vi "Begin.vi"(11 "Image Size":T1=enum."320x240") -> (0 "error out":errorcluster)   [LabVIEW 2012]
doc: "Called before other user functions, this VI is expected to open initial I/O refnums, load in file data, and do all program initialization. Notice that the <B>error out</B> terminal is simply used for data flow. Wiring it to other structures or subVIs ensures that this VI runs first."
uses:
  <vilib>/Rock Robotics/WPI/Camera/WPI_CameraImageSize.ctl
  <vilib>/Rock Robotics/WPI/DriverStation/WPI_DriverStationRobotMode2.ctl
  <vilib>/Rock Robotics/SystemInterfaces/DIO/FPGA_DIOPWMChannel.ctl
  <vilib>/Rock Robotics/WPI/Joystick/WPI_JoystickDeviceEnum.ctl
  <vilib>/Rock Robotics/SystemInterfaces/Typedef/FPGA_TypedefDigitalModule.ctl
  <vilib>/Rock Robotics/WPI/Relay/WPI_RelayDirection.ctl
  <vilib>/Rock Robotics/SystemInterfaces/DIO/FPGA_DIORelayChannel.ctl
  <vilib>/Rock Robotics/SystemInterfaces/AI/FPGA_AIChannel.ctl
  <vilib>/Rock Robotics/SystemInterfaces/AI/FPGA_AIGyroChannel.ctl
  <vilib>/Rock Robotics/SystemInterfaces/DIO/FPGA_DIOChannel.ctl
  <vilib>/Rock Robotics/WPI/Camera/WPI_CameraFrameRate.ctl
  Robot Global Data.vi
  <vilib>/Rock Robotics/WPI/MotorControl/WPI_MotorControlOpen Victor.vi
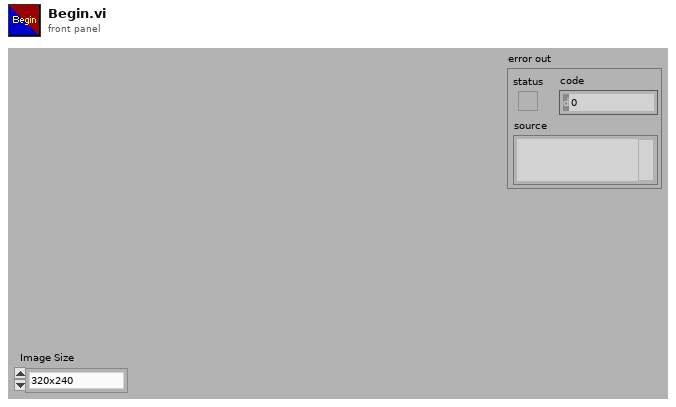
[diagram p1: front panel]
types:
  T1 = typedef "WPI_CameraImageSize.ctl" = enum16{"640x480", "320x240", "160x120"}
  T2 = typedef "FPGA_DIOChannel.ctl" = enum8{"DIO 1", "DIO 2", "DIO 3", "DIO 4", "DIO 5", "DIO 6", "DIO 7", "DIO 8", "DIO 9", "DIO 10", "DIO 11", "DIO 12", "DIO 13", "DIO 14", "Invalid"}
  T3 = typedef "FPGA_TypedefDigitalModule.ctl" = enum16{"Digital Module 1", "Digital Module 2"}
  T4 = typedef "FPGA_DIOPWMChannel.ctl" = enum8{"PWM 1", "PWM 2", "PWM 3", "PWM 4", "PWM 5", "PWM 6", "PWM 7", "PWM 8", "PWM 9", "PWM 10", "Invalid"}
  T5 = typedef "FPGA_DIORelayChannel.ctl" = enum8{"Relay 1", "Relay 2", "Relay 3", "Relay 4", "Relay 5", "Relay 6", "Relay 7", "Relay 8", "Invalid"}
  T6 = typedef "WPI_RelayDirection.ctl" = enum16{"Both directions", "Forward only", "Reverse only"}
  T7 = typedef "WPI_CameraFrameRate.ctl" = u32
  T8 = typedef "FPGA_AIChannel.ctl" = enum8{"AI 1", "AI 2", "AI 3", "AI 4", "AI 5", "AI 6", "AI 7", "AI 8", "Invalid"}
  T9 = typedef "FPGA_AIGyroChannel.ctl" = enum8{"AI 1", "AI 2", "Invalid"}
  T10 = typedef "WPI_JoystickDeviceEnum.ctl" = enum16{"USB 1", "USB 2", "USB 3", "USB 4", "Kinect 1", "Kinect 2"}
  T11 = typedef "WPI_DriverStationRobotMode2.ctl" = enum16{"Autonomous Disabled", "Autonomous Enabled", "Teleop Disabled", "Teleop Enabled", "Timeout", "Finish", "Test Disabled", "Test Enabled"}
  T12 = typedef "WPI_RelayDevRef.ctl" = cluster{"DevStatus":errorcluster, "Relay Channel":T5, "Digital Module":T3, "Relay Direction":T6}
  T13 = typedef "WPI_MotorControlDeviceRef.ctl" = cluster{"DeviceStatus":errorcluster, "Type":enum16{"PWM", "CAN"}, "PWM":cluster{"Digital Module":T3, "PWM Channel":T4, "DeadBand":T14}, "CAN":cluster{"Device Number":u8, "Control Mode":T15, "Semaphore":T16, "Max Vout":dbl}, "Invert":bool, "TransformRef":T17, "InvTransformRef":T17}
  T14 = typedef "WPI_PWMDeadband.ctl" = cluster{"Name":string, "maxPositivePwm":i32, "minPositivePwm":i32, "centerPwm":i32, "maxNegativePwm":i32, "minNegativePwm":i32, "angularRange":u16}
  T15 = typedef "WPI_CANJaguar_ControlMode.ctl" = enum8{"Percent VBus", "Current", "Speed", "Position", "Voltage"}
  T16 = typedef "Semaphore RefNum" = refnum<k1>
  T17 = typedef "WPI_PWMTransform_ConPane.ctl" = refnum<vi>
  T18 = typedef "WPI_JoystickDevRef.ctl" = cluster{"Device":T10}
  T19 = typedef "WPI_CameraDevRef.ctl" = cluster{"Camera Address":string, "CameraStatus":errorcluster, "Acquire Image Notifier":refnum<notifier>}
  T20 = typedef "WPI_ServoDeviceRef.ctl" = cluster{"DeviceStatus":errorcluster, "Digital Module":T3, "PWM Channel":T4, "DeadBand":T14}
  T21 = typedef "WPI_DigitalInputDevRef.ctl" = cluster{"DevStatus":errorcluster, "DIO Channel":T2, "Digital Module":T3}
  T22 = typedef "WPI_AnalogChannelDevRef.ctl" = cluster{"DevStatus":errorcluster, "Analog Module":T23, "Analog Channel":T8}
  T23 = typedef "FPGA_TypedefAnalogModule.ctl" = enum16{"Analog Module 1", "Analog Module 2"}
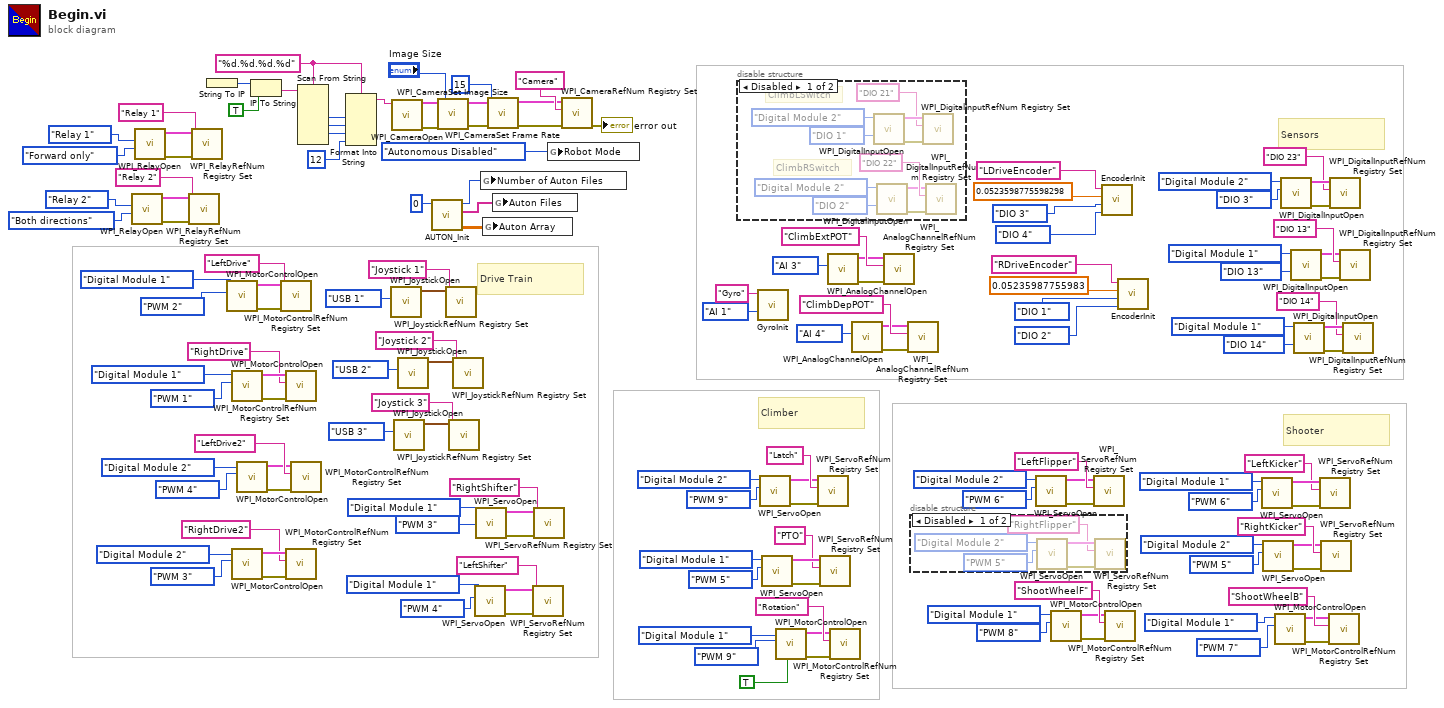
[diagram p0: block diagram]
diagram:
  w60 = "%d.%d.%d.%d" ("format string")
  # "Shooter"
  # "Drive Train"
  # "Climber"
  # "Sensors"
  n1 = call <vilib>:"WPI_RelayOpen.vi"("Relay Direction"=WPI_RelayDirection."Both directions", "Relay Channel"=FPGA_DIORelayChannel."Relay 2") -> ("error out"=w109:errorcluster, "RelayDevRef"=w110:T12)  [unwired: 8 in]
  n2 = call <vilib>:"WPI_RelayOpen.vi"("Relay Direction"=WPI_RelayDirection."Forward only", "Relay Channel"=FPGA_DIORelayChannel."Relay 1") -> ("error out"=w50:errorcluster, "RelayDevRef"=w49:T12)  [unwired: 8 in]
  n3 = call <vilib>:"WPI_RelayRefNum Registry Set.vi"("error in (no error)"=w109, "refnum name"="Relay 2", "RelayDevRef"=w110) -> ()  [unwired: 7 in, 2 out]
  n4 = call <vilib>:"WPI_RelayRefNum Registry Set.vi"("error in (no error)"=w50, "refnum name"="Relay 1", "RelayDevRef"=w49) -> ()  [unwired: 7 in, 2 out]
  n5 = String To IP() -> (0:w67:u32)  [unwired: 1 in]
  n6 = call-poly <vilib>:"WPI_MotorControlOpen.vi"("PWM Channel"=FPGA_DIOPWMChannel."PWM 2", "Digital Module (Module 1)"=FPGA_TypedefDigitalModule."Digital Module 1") -> ("error out"=w135:errorcluster, "MotorControlDeviceRef"=w136:T13)  [unwired: 8 in]
  n7 = call-poly <vilib>:"WPI_MotorControlOpen.vi"("PWM Channel"=FPGA_DIOPWMChannel."PWM 1", "Digital Module (Module 1)"=FPGA_TypedefDigitalModule."Digital Module 1") -> ("error out"=w142:errorcluster, "MotorControlDeviceRef"=w141:T13)  [unwired: 8 in]
  n8 = call-poly <vilib>:"WPI_MotorControlOpen.vi"("PWM Channel"=FPGA_DIOPWMChannel."PWM 3", "Digital Module (Module 1)"=FPGA_TypedefDigitalModule."Digital Module 2") -> ("error out"=w124:errorcluster, "MotorControlDeviceRef"=w123:T13)  [unwired: 8 in]
  n9 = call-poly <vilib>:"WPI_MotorControlOpen.vi"("PWM Channel"=FPGA_DIOPWMChannel."PWM 4", "Digital Module (Module 1)"=FPGA_TypedefDigitalModule."Digital Module 2") -> ("error out"=w115:errorcluster, "MotorControlDeviceRef"=w116:T13)  [unwired: 8 in]
  n10 = IP To String(1:TRUE ("dot notation? (F)"), 2:w67) -> (0:w65:string)
  n11 = call <vilib>:"WPI_MotorControlRefNum Registry Set.vi"("error in (no error)"=w135, "refnum name"="LeftDrive", "MotorControlDevRef"=w136) -> ()  [unwired: 7 in, 2 out]
  n12 = call <vilib>:"WPI_MotorControlRefNum Registry Set.vi"("error in (no error)"=w142, "refnum name"="RightDrive", "MotorControlDevRef"=w141) -> ()  [unwired: 7 in, 2 out]
  n13 = call <vilib>:"WPI_MotorControlRefNum Registry Set.vi"("error in (no error)"=w124, "refnum name"="RightDrive2", "MotorControlDevRef"=w123) -> ()  [unwired: 7 in, 2 out]
  n14 = call <vilib>:"WPI_MotorControlRefNum Registry Set.vi"("error in (no error)"=w115, "refnum name"="LeftDrive2", "MotorControlDevRef"=w116) -> ()  [unwired: 7 in, 2 out]
  n15 = Scan From String(format string=w60, input string=w65) -> (output 1=w64:i32, output 2=w63:i32, output 3=w62:i32)  [unwired: 7 in, 3 out]
  n16 = Format Into String(format string=w60, w64, w63, w62, 12 ("Compression")) -> (resulting string=w59:string)  [unwired: 2 in, 1 out]
  n17 = call <vilib>:"WPI_JoystickOpen.vi"("JoystickDevice"=WPI_JoystickDeviceEnum."USB 1") -> ("JoystickDevRef"=w126:T18)  [unwired: 10 in]
  n18 = call <vilib>:"WPI_CameraOpen.vi"("Camera Address"=w59) -> ("error out"=w58:errorcluster, "CameraDevRef"=w57:T19)  [unwired: 1 in, 8 out]
  n19 = call <vilib>:"WPI_JoystickOpen.vi"("JoystickDevice"=WPI_JoystickDeviceEnum."USB 3") -> ("JoystickDevRef"=w132:T18)  [unwired: 10 in]
  n20 = call <vilib>:"WPI_JoystickOpen.vi"("JoystickDevice"=WPI_JoystickDeviceEnum."USB 2") -> ("JoystickDevRef"=w131:T18)  [unwired: 10 in]
  n21 = call "AUTON_Init.vi"("Default File"=0) -> ("Auton Array"=w143:dbl[][], "Auton Files"=w144:string[], "Number of Auton Files"=w145:i64)  [unwired: 8 in]
  n22 = call <vilib>:"WPI_CameraSet Image Size.vi"("error in (no error)"=w58, "Image Size"="Image Size", "CameraDevRef"=w57) -> ("error out"=w55:errorcluster, "CameraDevRef Out"=w56:T19)  [unwired: 7 out]
  n23 = call <vilib>:"WPI_JoystickRefNum Registry Set.vi"("refnum name"="Joystick 1", "JoystickDevRef"=w126) -> ()  [unwired: 8 in, 2 out]
  n24 = call <vilib>:"WPI_JoystickRefNum Registry Set.vi"("refnum name"="Joystick 3", "JoystickDevRef"=w132) -> ()  [unwired: 8 in, 2 out]
  n25 = call <vilib>:"WPI_JoystickRefNum Registry Set.vi"("refnum name"="Joystick 2", "JoystickDevRef"=w131) -> ()  [unwired: 8 in, 2 out]
  n26 = call <vilib>:"WPI_ServoOpen.vi"("PWM Channel"=FPGA_DIOPWMChannel."PWM 4", "Digital Module (Module 1)"=FPGA_TypedefDigitalModule."Digital Module 1") -> ("error out"=w108:errorcluster, "ServoDeviceRef"=w101:T20)  [unwired: 8 in]
  n27 = call <vilib>:"WPI_ServoOpen.vi"("PWM Channel"=FPGA_DIOPWMChannel."PWM 3", "Digital Module (Module 1)"=FPGA_TypedefDigitalModule."Digital Module 1") -> ("error out"=w107:errorcluster, "ServoDeviceRef"=w106:T20)  [unwired: 8 in]
  n28 = global write "Robot Global Data.vi" "Number of Auton Files"(w145) -> ()
  n29 = global write "Robot Global Data.vi" "Auton Array"(w143) -> ()
  n30 = call <vilib>:"WPI_CameraSet Frame Rate.vi"("error in (no error)"=w55, "Frame Rate (fps)"=T7 15, "CameraDevRef"=w56) -> ("error out"=w54:errorcluster, "CameraDevRef Out"=w53:T19)  [unwired: 7 out]
  n31 = global write "Robot Global Data.vi" "Auton Files"(w144) -> ()
  n32 = call <vilib>:"WPI_ServoRefNum Registry Set.vi"("error in (no error)"=w108, "refnum name"="LeftShifter", "ServoDeviceRef"=w101) -> ()  [unwired: 7 in, 2 out]
  n33 = call <vilib>:"WPI_ServoRefNum Registry Set.vi"("error in (no error)"=w107, "refnum name"="RightShifter", "ServoDeviceRef"=w106) -> ()  [unwired: 7 in, 2 out]
  n34 = global write "Robot Global Data.vi" "Robot Mode"(WPI_DriverStationRobotMode2."Autonomous Disabled" ("Robot Mode")) -> ()
  n35 = call <vilib>:"WPI_CameraRefNum Registry Set.vi"("error in (no error)"=w54, "refnum name"="Camera", "CameraDevRef"=w53) -> ("error out"=→"error out":errorcluster)  [unwired: 8 out]
  n36 = disable-structure shown="Disabled" {
    frame Disabled {
      # "ClimbRSwitch"
      # "ClimbLSwitch"
      n37 = call <vilib>:"WPI_DigitalInputOpen.vi"("DIO Channel"=FPGA_DIOChannel."DIO 1", "Digital Module (Module 1)"=FPGA_TypedefDigitalModule."Digital Module 2") -> ("error out"=w149:errorcluster, "DigitalInputDevRef"=w150:T21)  [unwired: 8 in]
      n38 = call <vilib>:"WPI_DigitalInputOpen.vi"("DIO Channel"=FPGA_DIOChannel."DIO 2", "Digital Module (Module 1)"=FPGA_TypedefDigitalModule."Digital Module 2") -> ("error out"=w156:errorcluster, "DigitalInputDevRef"=w155:T21)  [unwired: 8 in]
      n39 = call <vilib>:"WPI_DigitalInputRefNum Registry Set.vi"("error in (no error)"=w149, "refnum name"="DIO 21", "DigitalInputDevRef"=w150) -> ()  [unwired: 7 in, 2 out]
      n40 = call <vilib>:"WPI_DigitalInputRefNum Registry Set.vi"("error in (no error)"=w156, "refnum name"="DIO 22", "DigitalInputDevRef"=w155) -> ()  [unwired: 7 in, 2 out]
    }
    frame Enabled {
    }
  }
  n41 = call "GyroInit.vi"("refnum name"="Gyro", "Analog Channel"=FPGA_AIGyroChannel."AI 1") -> ()  [unwired: 8 in]
  n42 = call <vilib>:"WPI_ServoOpen.vi"("PWM Channel"=FPGA_DIOPWMChannel."PWM 9", "Digital Module (Module 1)"=FPGA_TypedefDigitalModule."Digital Module 2") -> ("error out"=w42:errorcluster, "ServoDeviceRef"=w43:T20)  [unwired: 8 in]
  n43 = call <vilib>:"WPI_ServoOpen.vi"("PWM Channel"=FPGA_DIOPWMChannel."PWM 5", "Digital Module (Module 1)"=FPGA_TypedefDigitalModule."Digital Module 1") -> ("error out"=w86:errorcluster, "ServoDeviceRef"=w85:T20)  [unwired: 8 in]
  n44 = call-poly <vilib>:"WPI_MotorControlOpen.vi"("Invert"=TRUE, "PWM Channel"=FPGA_DIOPWMChannel."PWM 9", "Digital Module (Module 1)"=FPGA_TypedefDigitalModule."Digital Module 1") -> ("error out"=w91:errorcluster, "MotorControlDeviceRef"=w90:T13)  [unwired: 7 in]
  n45 = call <vilib>:"WPI_ServoRefNum Registry Set.vi"("error in (no error)"=w42, "refnum name"="Latch", "ServoDeviceRef"=w43) -> ()  [unwired: 7 in, 2 out]
  n46 = call <vilib>:"WPI_ServoRefNum Registry Set.vi"("error in (no error)"=w86, "refnum name"="PTO", "ServoDeviceRef"=w85) -> ()  [unwired: 7 in, 2 out]
  n47 = call <vilib>:"WPI_AnalogChannelOpen.vi"("Analog Channel"=FPGA_AIChannel."AI 3") -> ("error out"=w70:errorcluster, "AIDeviceRef"=w71:T22)  [unwired: 9 in]
  n48 = call <vilib>:"WPI_MotorControlRefNum Registry Set.vi"("error in (no error)"=w91, "refnum name"="Rotation", "MotorControlDevRef"=w90) -> ()  [unwired: 7 in, 2 out]
  n49 = call <vilib>:"WPI_AnalogChannelOpen.vi"("Analog Channel"=FPGA_AIChannel."AI 4") -> ("error out"=w95:errorcluster, "AIDeviceRef"=w96:T22)  [unwired: 9 in]
  n50 = call <vilib>:"WPI_AnalogChannelRefNum Registry Set.vi"("error in (no error)"=w70, "refnum name"="ClimbExtPOT", "AIDeviceRef"=w71) -> ()  [unwired: 7 in, 2 out]
  n51 = call <vilib>:"WPI_AnalogChannelRefNum Registry Set.vi"("error in (no error)"=w95, "refnum name"="ClimbDepPOT", "AIDeviceRef"=w96) -> ()  [unwired: 7 in, 2 out]
  n52 = disable-structure shown="Disabled" {
    frame Disabled {
      n53 = call <vilib>:"WPI_ServoOpen.vi"("PWM Channel"=FPGA_DIOPWMChannel."PWM 5", "Digital Module (Module 1)"=FPGA_TypedefDigitalModule."Digital Module 2") -> ("error out"=w162:errorcluster, "ServoDeviceRef"=w161:T20)  [unwired: 8 in]
      n54 = call <vilib>:"WPI_ServoRefNum Registry Set.vi"("error in (no error)"=w162, "refnum name"="RightFlipper", "ServoDeviceRef"=w161) -> ()  [unwired: 7 in, 2 out]
    }
    frame Enabled {
    }
  }
  n55 = call <vilib>:"WPI_ServoOpen.vi"("PWM Channel"=FPGA_DIOPWMChannel."PWM 6", "Digital Module (Module 1)"=FPGA_TypedefDigitalModule."Digital Module 2") -> ("error out"=w26:errorcluster, "ServoDeviceRef"=w27:T20)  [unwired: 8 in]
  n56 = call-poly <vilib>:"WPI_MotorControlOpen.vi"("PWM Channel"=FPGA_DIOPWMChannel."PWM 8", "Digital Module (Module 1)"=FPGA_TypedefDigitalModule."Digital Module 1") -> ("error out"=w37:errorcluster, "MotorControlDeviceRef"=w38:T13)  [unwired: 8 in]
  n57 = call <vilib>:"WPI_ServoRefNum Registry Set.vi"("error in (no error)"=w26, "refnum name"="LeftFlipper", "ServoDeviceRef"=w27) -> ()  [unwired: 7 in, 2 out]
  n58 = call "EncoderInit.vi"("refnum name"="LDriveEncoder", "DistancePerCount"=0.0523598775598298, "DIO Channel"=FPGA_DIOChannel."DIO 3", "DIO Channel 2"=FPGA_DIOChannel."DIO 4") -> ()  [unwired: 7 in]
  n59 = call <vilib>:"WPI_MotorControlRefNum Registry Set.vi"("error in (no error)"=w37, "refnum name"="ShootWheelF", "MotorControlDevRef"=w38) -> ()  [unwired: 7 in, 2 out]
  n60 = call "EncoderInit.vi"("refnum name"="RDriveEncoder", "DistancePerCount"=0.05235987755983, "DIO Channel"=FPGA_DIOChannel."DIO 1", "DIO Channel 2"=FPGA_DIOChannel."DIO 2") -> ()  [unwired: 7 in]
  n61 = call <vilib>:"WPI_ServoOpen.vi"("PWM Channel"=FPGA_DIOPWMChannel."PWM 6", "Digital Module (Module 1)"=FPGA_TypedefDigitalModule."Digital Module 1") -> ("error out"=w21:errorcluster, "ServoDeviceRef"=w20:T20)  [unwired: 8 in]
  n62 = call <vilib>:"WPI_ServoOpen.vi"("PWM Channel"=FPGA_DIOPWMChannel."PWM 5", "Digital Module (Module 1)"=FPGA_TypedefDigitalModule."Digital Module 2") -> ("error out"=w16:errorcluster, "ServoDeviceRef"=w22:T20)  [unwired: 8 in]
  n63 = call-poly <vilib>:"WPI_MotorControlOpen.vi"("PWM Channel"=FPGA_DIOPWMChannel."PWM 7", "Digital Module (Module 1)"=FPGA_TypedefDigitalModule."Digital Module 1") -> ("error out"=w33:errorcluster, "MotorControlDeviceRef"=w32:T13)  [unwired: 8 in]
  n64 = call <vilib>:"WPI_DigitalInputOpen.vi"("DIO Channel"=FPGA_DIOChannel."DIO 3", "Digital Module (Module 1)"=FPGA_TypedefDigitalModule."Digital Module 2") -> ("error out"=w1:errorcluster, "DigitalInputDevRef"=w4:T21)  [unwired: 8 in]
  n65 = call <vilib>:"WPI_DigitalInputOpen.vi"("DIO Channel"=FPGA_DIOChannel."DIO 13", "Digital Module (Module 1)"=FPGA_TypedefDigitalModule."Digital Module 1") -> ("error out"=w14:errorcluster, "DigitalInputDevRef"=w13:T21)  [unwired: 8 in]
  n66 = call <vilib>:"WPI_DigitalInputOpen.vi"("DIO Channel"=FPGA_DIOChannel."DIO 14", "Digital Module (Module 1)"=FPGA_TypedefDigitalModule."Digital Module 1") -> ("error out"=w7:errorcluster, "DigitalInputDevRef"=w8:T21)  [unwired: 8 in]
  n67 = call <vilib>:"WPI_ServoRefNum Registry Set.vi"("error in (no error)"=w21, "refnum name"="LeftKicker", "ServoDeviceRef"=w20) -> ()  [unwired: 7 in, 2 out]
  n68 = call <vilib>:"WPI_ServoRefNum Registry Set.vi"("error in (no error)"=w16, "refnum name"="RightKicker", "ServoDeviceRef"=w22) -> ()  [unwired: 7 in, 2 out]
  n69 = call <vilib>:"WPI_MotorControlRefNum Registry Set.vi"("error in (no error)"=w33, "refnum name"="ShootWheelB", "MotorControlDevRef"=w32) -> ()  [unwired: 7 in, 2 out]
  n70 = call <vilib>:"WPI_DigitalInputRefNum Registry Set.vi"("error in (no error)"=w1, "refnum name"="DIO 23", "DigitalInputDevRef"=w4) -> ()  [unwired: 7 in, 2 out]
  n71 = call <vilib>:"WPI_DigitalInputRefNum Registry Set.vi"("error in (no error)"=w14, "refnum name"="DIO 13", "DigitalInputDevRef"=w13) -> ()  [unwired: 7 in, 2 out]
  n72 = call <vilib>:"WPI_DigitalInputRefNum Registry Set.vi"("error in (no error)"=w7, "refnum name"="DIO 14", "DigitalInputDevRef"=w8) -> ()  [unwired: 7 in, 2 out]
